vi "Pulse duration analysis.vi"() -> ()   [LabVIEW 2015]
uses:
  ESA_Data_Analysis_Global_VIs.vi
  <vilib>/Analysis/3filter.llb/Butterworth Filter (DBL).vi
  <vilib>/Analysis/NI_AALBase.lvlib
panel:
  out "Waveform Graph 2":dbl[](graph)
  out "Waveform Graph":dbl[](graph)
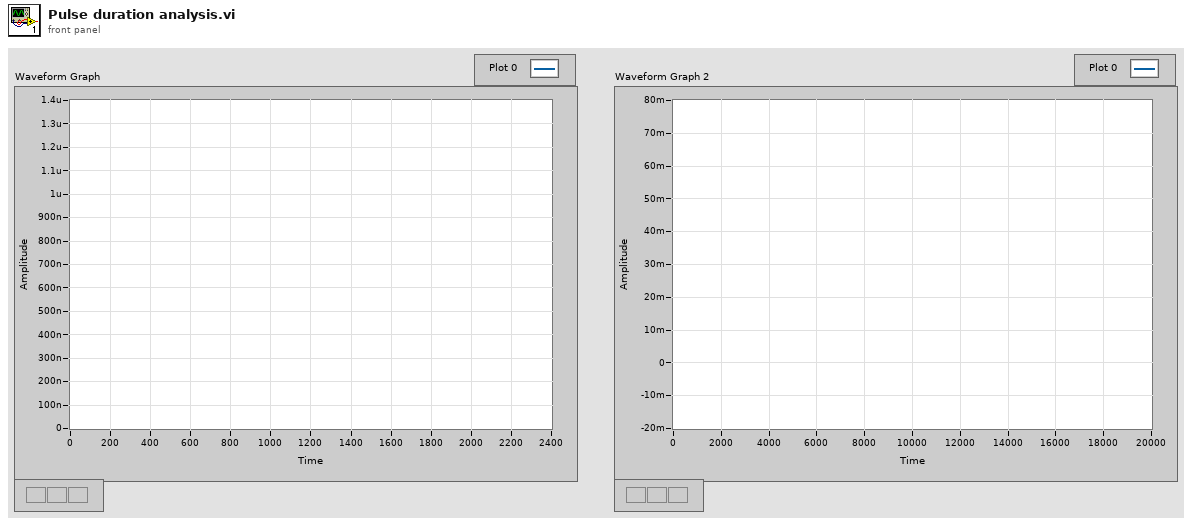
[diagram p1: front panel]
types:
  T1 = cluster{"Cursor.Cursor X1":dbl, "Cursor.Cursor Y1":dbl, "Cursor.Cursor X2":dbl, "Cursor.Cursor Y2":dbl}
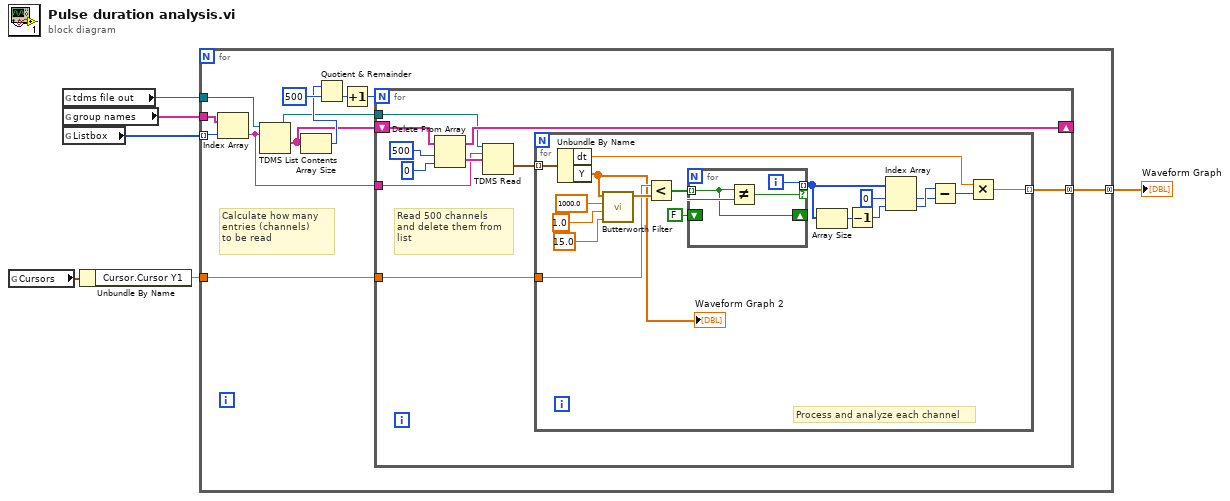
[diagram p0: block diagram]
diagram:
  n1 = global read "ESA_Data_Analysis_Global_VIs.vi" "Cursors"() -> (w3:T1)
  n2 = global read "ESA_Data_Analysis_Global_VIs.vi" "tdms file out"() -> (w6:refnum<k34>)
  n3 = global read "ESA_Data_Analysis_Global_VIs.vi" "group names"() -> (w5:string[])
  n4 = global read "ESA_Data_Analysis_Global_VIs.vi" "Listbox"() -> (w4:i32[])
  n5 = Unbundle By Name(w3) -> ("Cursor.Cursor Y1"=w2:dbl)
  n6 = for {
    tunnel: w6 -> [w18]
    tunnel: w5 -> [w17]
    tunnel: w4 -> [w16] mode=indexing
    tunnel: w2 -> [w8]
    tunnel: [w7] -> w1 mode=concatenating
    # "Calculate how many \nentries (channels) \nto be read"
    n7 = Index Array(array=w17, index=w16) -> (element=w10:string)
    n8 = TDMS List Contents(6:w10, 7:w18) -> (1:w11:string[], 3:w9:refnum<k34>)  [unwired: 1 in, 2 out]
    n9 = Array Size(array=w11) -> (size(s)=w12:i32)
    n10 = Quotient & Remainder(x=w12, y=500) -> (floor(x/y)=w14:i32)  [unwired: 1 out]
    n11 = Increment(x=w14) -> (x+1=w13:i32)
    n12 = for {
      N: w13 -> [_]
      shift-right: [w23] -> _
      shift-left: w11 -> [w26]
      tunnel: w10 -> [w24]
      tunnel: w9 -> [w21]
      tunnel: w8 -> [w20]
      tunnel: [w19] -> w7 mode=concatenating
      # "Read 500 channels\nand delete them from\nlist"
      n13 = Delete From Array(array=w26, length=500, index=0) -> (deleted portion=w25:string[], array with subset deleted=w23:string[])
      n14 = TDMS Read(0:w21, 5:w24, 7:w25) -> (10:w22:waveform(dbl)[])  [unwired: 5 in, 5 out]
      n15 = for {
        tunnel: w22 -> [w46] mode=indexing
        tunnel: w20 -> [w41]
        tunnel: [w30] -> w19 mode=indexing
        # "Process and analyze each channel"
        n16 = Unbundle By Name(w46) -> ("dt"=w31:dbl, "Y"=w29:dbl[])
        "Waveform Graph 2" <- w29
        n17 = call-poly <vilib>:"Butterworth Filter.vi"("low cutoff freq: fl"=15.0, "high cutoff freq: fh"=1.0, "sampling freq: fs"=1000.0, "X"=w29) -> ("Filtered X"=w42:dbl[])  [unwired: 4 in, 1 out]
        n18 = Less?(x=w41, y=w42) -> (x < y?=w40:bool[])
        n19 = for {
          tunnel: w40 -> [w49] mode=indexing
          shift-right: [w49] -> _
          shift-left: FALSE -> [w50]
          tunnel: [w47] -> w37 mode=indexing if=w48
          i -> [w47]
          n20 = Not Equal?(x=w49, y=w50) -> (x != y?=w48:bool)
        }
        n21 = Array Size(array=w37) -> (size(s)=w36:i32)
        n22 = Decrement(x=w36) -> (x-1=w35:i32)
        n23 = Index Array(array=w37, index #1=0 ("index"), index #2=w35) -> (element #1=w33:i32, element #2=w34:i32)
        n24 = Subtract(x=w34, y=w33) -> (x-y=w32:i32)
        n25 = Multiply(x=w31, y=w32) -> (x*y=w30:dbl)
      }
    }
  }
  "Waveform Graph" <- w1
